vi "LVObject to JSON - Object With Member - Returns JSON Object With Member.vi"() -> ()   [LabVIEW 2017, in "Tests.lvlib"]
uses:
  Tests.lvlib
  Flatten To JSON Object/Flatten To JSON Object.lvclass
  Weather Forecast/Weather Forecast.lvclass
  <vilib>/addons/_JKI Toolkits/Caraya/classes/Assert/Assert Equal Value_Variant.vi
  <vilib>/addons/_JKI Toolkits/Caraya/classes/Test/Test.lvclass
  <vilib>/addons/_JKI Toolkits/Caraya/classes/Assert/Assert.lvclass
panel:
  out "error out":errorcluster
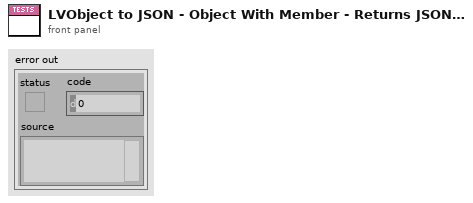
[diagram p1: front panel]
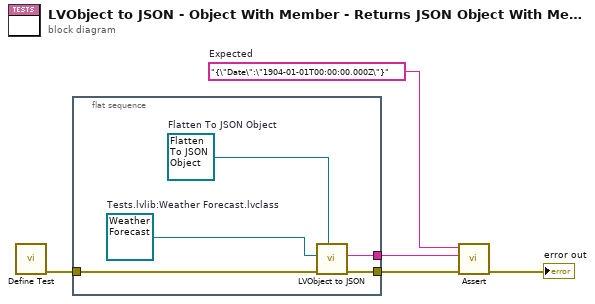
[diagram p0: block diagram]
diagram:
  w1 = "{\"Date\":\"1904-01-01T00:00:00.000Z\"}"  # Expected
  n1 = call <vilib>:"Define Test.vi"() -> ("error out"=w4:errorcluster)  [unwired: 11 in]
  n2 = flat-sequence {
    tunnel: w4 -> [w9]
    tunnel: [w8] -> w3
    tunnel: [w6] -> w2
    frame #0 {
      w7 = refnum<class "Weather Forecast.lvclass"> refnum  # Tests.lvlib:Weather Forecast.lvclass
      w10 = refnum<class "Flatten To JSON Object.lvclass"> refnum  # Flatten To JSON Object
      n3 = call-dynamic "LVObject to JSON.vi"("Flatten To JSON Object in"=w10, "error in (no error)"=w9, "Object"=w7) -> ("error out"=w8:errorcluster, "<JSON>Object"=w6:string)  [unwired: 7 in]
    }
  }
  n4 = call-poly <vilib>:"Assert.vi"("error in (no error)"=w3, "Y"=w2, "X"=w1) -> ("error out"=→"error out":errorcluster)  [unwired: 8 in]
